vi "Get Channel Information.vi"(9 "FPGA Name":string, 10 "Channel Type":string, 11 "myRIO PID":string) -> (2 "Pin Info":string[][](array[string]), 3 "Channel List":string[](array[string]))   [LabVIEW 2021]
uses:
  <vilib>/myRIO/Common/Instrument Driver Framework/Utilities/typedefs/Channel Types.ctl
  <vilib>/myRIO/Common/Instrument Driver Framework/Utilities/typedefs/Pin Info List Array.ctl
  <vilib>/myRIO/Common/Instrument Driver Framework/Utilities/typedefs/Pin Info Cluster.ctl
  <vilib>/myRIO/Common/Instrument Driver Framework/Utilities/typedefs/Channel List Array.ctl
  <vilib>/myRIO/Common/Instrument Driver Framework/Utilities/typedefs/Channel List Cluster.ctl
  <vilib>/myRIO/Common/FPGA Personality Framework/Personality.lvlib
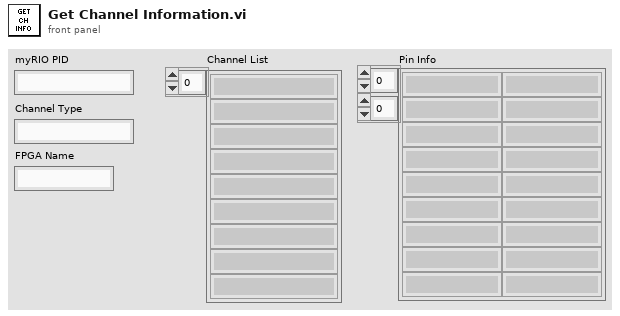
[diagram p1: front panel]
types:
  T1 = typedef "Channel Types.ctl" = enum32{"Unknown", "AI", "AO", "DIO - DI", "DIO", "DIO - DO", "I2C", "PWM", "Encoder", "SPI", "UART", "Accelerometer", "DIO - LED", "DIO - Button", "AI (N Samples)", "AudioIn (N Samples)", "AO (N Samples)", "AudioOut (N Samples)", "DI (N Samples)", "DO (N Samples)", "AI IRQ", "DI IRQ", "Timer IRQ", "RSL", "Relay", "CAN", "AI (Continuous)", "AO (Continuous)"}
  T2 = typedef "Pin Info List Array.ctl" = T3[]
  T3 = typedef "Pin Info Cluster.ctl" = cluster{"Pin Info":string[][]}
  T4 = typedef "Channel List Array.ctl" = T5[]
  T5 = typedef "Channel List Cluster.ctl" = cluster{"Channel List":string[]}
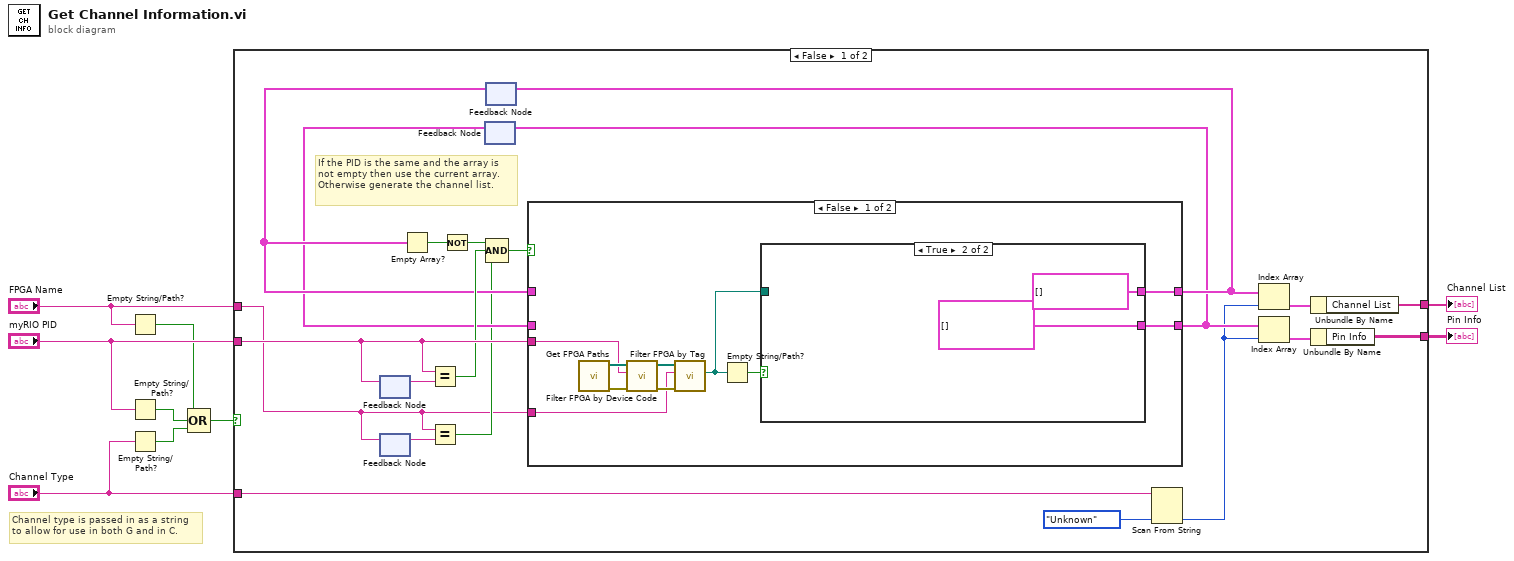
[diagram p0: block diagram]
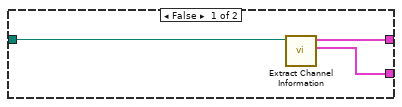
[diagram p2: hidden frame]
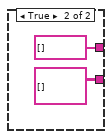
[diagram p4: hidden frame]
diagram:
  # "Channel type is passed in as a string\nto allow for use in both G and in C."
  n1 = Empty String/Path?(string/path="FPGA Name") -> (empty?=w1:bool)
  n2 = Empty String/Path?(string/path="myRIO PID") -> (empty?=w7:bool)
  n3 = Empty String/Path?(string/path="Channel Type") -> (empty?=w6:bool)
  n4 = Compound Arithmetic op=OR(w1, w7, w6) -> (w5:bool)
  n5 = case shown="False" w5 {
    tunnel: "myRIO PID" -> [w29 _]
    tunnel: "Channel Type" -> [w28 _]
    tunnel: [w14 string[] [] ("Channel List")] -> w9
    tunnel: [w13 string[][] [] ("Pin Info")] -> w8
    tunnel: "FPGA Name" -> [w10 _]
    frame False {
      # "If the PID is the same and the array is not empty then use the current array. Otherwise generate the channel list."
      n6 = feedback #1() -> (w25:string)  [unwired: 1 in]
      n7 = feedback-in #1(w29) -> ()
      n8 = feedback #2() -> (w12:string)  [unwired: 1 in]
      n9 = feedback-in #2(w10) -> ()
      n10 = Equal?(x=w29, y=w25) -> (x = y?=w24:bool)
      n11 = Equal?(x=w10, y=w12) -> (x = y?=w11:bool)
      n12 = feedback #3() -> (w19:T2)  [unwired: 1 in]
      n13 = feedback #4() -> (w20:T4)  [unwired: 1 in]
      n14 = Empty Array?(array=w20) -> (empty?=w23:bool)
      n15 = Not(x=w23) -> (.not. x?=w22:bool)
      n16 = Compound Arithmetic op=AND(w22, w24, w11) -> (w21:bool)
      n17 = case shown="False" w21 {
        tunnel: [w39 w46] -> w18
        tunnel: w20 -> [_ w46]
        tunnel: w29 -> [w31 _]
        tunnel: w19 -> [_ w45]
        tunnel: [w37 w45] -> w17
        tunnel: w10 -> [w30 _]
        frame False {
          n18 = call <vilib>:"Get FPGA Paths.vi"() -> ("error out"=w36:errorcluster, "FPGA Personality File Paths"=w33:path[])  [unwired: 10 in]
          n19 = call <vilib>:"Filter FPGA by Device Code.vi"("error in (no error)"=w36, "Device Code"=w31, "FPGA Personality File Paths"=w33) -> ("error out"=w35:errorcluster, "Filtered FPGA Personality File Paths"=w32:path[])  [unwired: 7 in]
          n20 = call <vilib>:"Filter FPGA by Tag.vi"("error in (no error)"=w35, "FPGA Personality Tag"=w30, "FPGA Personality File Paths"=w32) -> ("First Path"=w34:path)  [unwired: 6 in, 2 out]
          n21 = Empty String/Path?(string/path=w34) -> (empty?=w38:bool)
          n22 = case shown="True" w38 {
            tunnel: [w42 T4 [] ("Channel List")] -> w39
            tunnel: [w41 T2 [] ("Pin Info List")] -> w37
            tunnel: w34 -> [w40 _]
            frame False {
              n23 = call <vilib>:"Extract Channel Information.vi"("Channel Info File"=w40) -> ("Pin Info List"=w41:T2, "Channel List"=w42:T4)  [unwired: 9 in]
            }
            frame True {
            }
          }
        }
        frame True {
          # "Use the stored list"
        }
      }
      n24 = feedback-in #3(w17) -> ()
      n25 = feedback-in #4(w18) -> ()
      n26 = Scan From String(input string=w28, default 1=Channel_Types."Unknown" ("Channel Types")) -> (output 1=w16:T1)  [unwired: 3 in, 3 out]
      n27 = Index Array(array=w18, index=w16) -> (element=w26:T5)
      n28 = Index Array(array=w17, index=w16) -> (element=w15:T3)
      n29 = Unbundle By Name(w26) -> ("Channel List"=w14:string[])
      n30 = Unbundle By Name(w15) -> ("Pin Info"=w13:string[][])
    }
    frame True {
    }
  }
  "Channel List" <- w9
  "Pin Info" <- w8
